vi "Z Aux Modbus Get0x.vi"(7 "pdata":string, 8 "error in (no error)":errorcluster caption="错误输入（无错误）", 9 "inum":u16, 10 "start":u16, 11 "handle":u32) -> (0 "error out":errorcluster caption="错误输出", 2 "function return":i32, 3 "handle out":u32, 5 "pdata out":string)   [LabVIEW 2015, in "zauxdll.lvlib"]
doc: "int32 __stdcall ZAux_Modbus_Get0x(ZMC_HANDLE handle, uint16 start, uint16 inum, uint8 pdata[]);"
uses:
  zauxdll.lvlib
  Radar - 2015 32bit_autoqueue_angle_0319/zauxdll-2014/zauxdll.dll
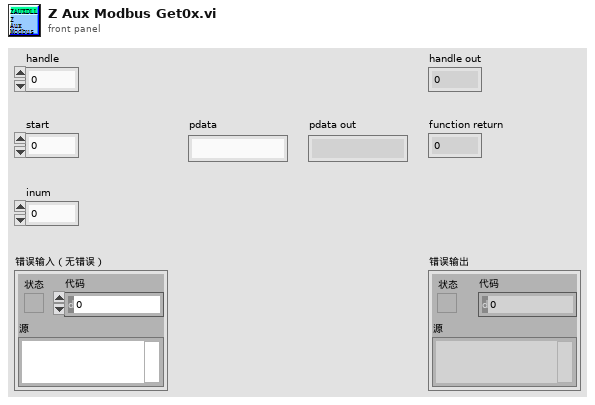
[diagram p1: front panel]
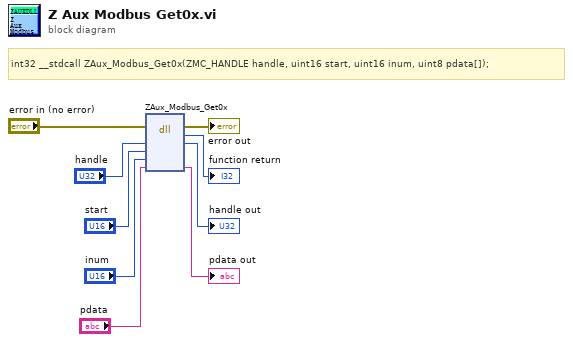
[diagram p0: block diagram]
diagram:
  # "int32 __stdcall ZAux_Modbus_Get0x(ZMC_HANDLE handle, uint16 start, uint16 inum, uint8 pdata[]);"
  n1 = dll-call lib="D:/vicomm case/cub/0717/Radar - 2015 32bit_autoqueue_angle_0319/zauxdll-2014/zauxdll.*" fn="ZAux_Modbus_Get0x"(error in="error in (no error)", "handle"="handle", "start"="start", "inum"="inum", "pdata"="pdata") -> (error out=→"error out":errorcluster, →"function return":i32, "handle"=→"handle out":u32, "pdata"=→"pdata out":string)  [unwired: 4 in, 1 out]
